vi "ValidateExpression.vi"(8 "error in (no error)":errorcluster, 10 "Expression":string, 11 "Cron in":refnum<class "Cron.lvclass">) -> (0 "error out":errorcluster, 1 "valid?":bool, 2 "Expression dup":string, 3 "Cron out":refnum<class "Cron.lvclass">)   [LabVIEW 2013, in "openCron.lvlib" / "Cron.lvclass"]
uses:
  Cron.lvclass
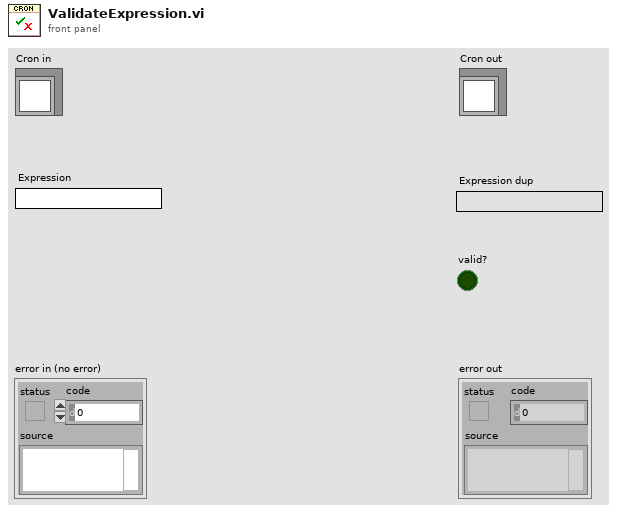
[diagram p1: front panel]
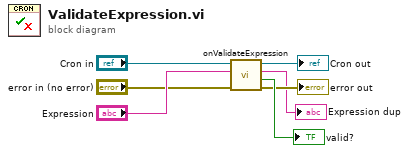
[diagram p0: block diagram]
diagram:
  n1 = call-dynamic "onValidateExpression.vi"("error in (no error)"="error in (no error)", "Expression"="Expression", "Cron in"="Cron in") -> ("error out"=→"error out":errorcluster, "valid?"=→"valid?":bool, "Validated Expression"=→"Expression dup":string, "Cron out"=→"Cron out":refnum<class "Cron.lvclass">)  [unwired: 5 in]
